vi "ON-OFF Cycle Timer - msec (SubVI).vi"(0 "ENABLE OUTPUT":bool, 5 "START/RESET":bool, 7 "ON Time [ms]":u32=10, 9 "OFF Time [ms]":u32=10, 11 "Cycle Limit":i32=100 min=-1) -> (4 "OUTPUT":bool, 6 "Cycle Change":bool, 8 "Cycles Complete":bool, 10 "Total Elapsed Time [ms]":u32, 14 "Display":string, 15 "Cycle Count":i32)   [LabVIEW 2012]
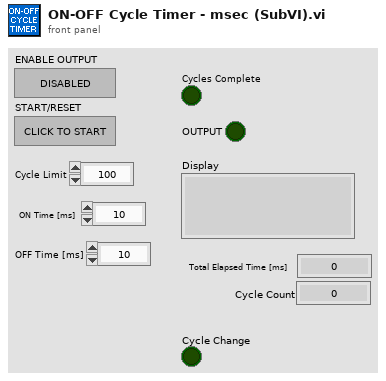
[diagram p1: front panel]
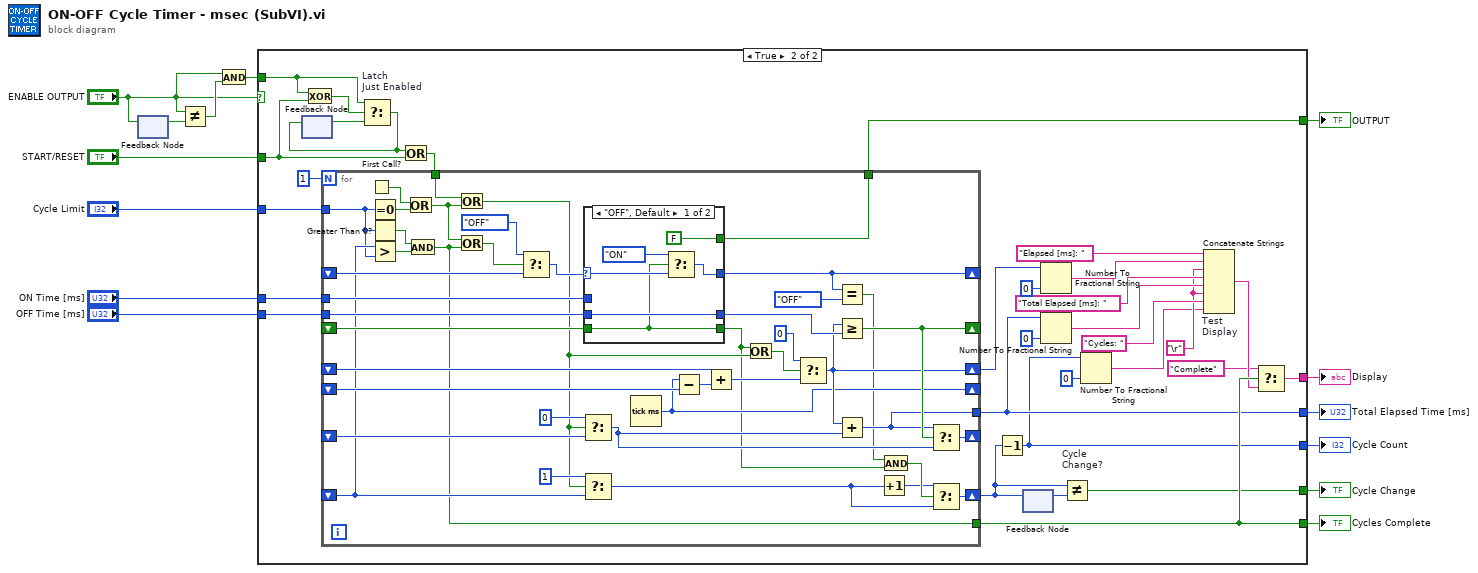
[diagram p0: block diagram]
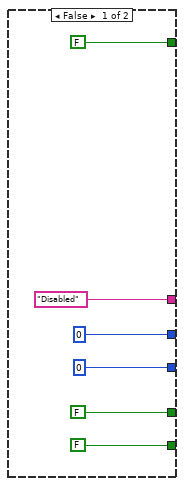
[diagram p2: hidden frame]
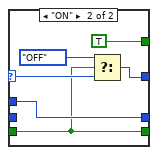
[diagram p3: hidden frame]
diagram:
  n1 = feedback #1() -> (w10:bool)  [unwired: 1 in]
  n2 = feedback-in #1("ENABLE OUTPUT") -> ()
  n3 = Not Equal?(x="ENABLE OUTPUT", y=w10) -> (x != y?=w12:bool)
  n4 = And(x="ENABLE OUTPUT", y=w12) -> (x .and. y?=w13:bool)
  n5 = case shown="True" "ENABLE OUTPUT" {
    tunnel: "ON Time [ms]" -> [_ w51]
    tunnel: "OFF Time [ms]" -> [_ w50]
    tunnel: [FALSE w38] -> w3
    tunnel: [FALSE w33] -> w4
    tunnel: [u32 0 w32] -> w5
    tunnel: [0 w31] -> w6
    tunnel: "Cycle Limit" -> [_ w28]
    tunnel: [FALSE w30] -> w8
    tunnel: ["Disabled" w29] -> w9
    tunnel: w13 -> [_ w25]
    tunnel: "START/RESET" -> [_ w23]
    frame False {
    }
    frame True {
      w41 = "\r"
      n6 = feedback #2() -> (w27:bool)  [unwired: 1 in]
      n7 = Exclusive Or(1:w23, 2:w25) -> (0:w26:bool)
      n8 = Select "Latch\nJust Enabled"(t=w25, s=w26, f=w27) -> (s? t:f=w24:bool)
      n9 = feedback-in #2(w24) -> ()
      n10 = Or(x=w24, y=w23) -> (x .or. y?=w22:bool)
      n11 = for {
        N: 1 -> [_]
        shift-right: [w78] -> _
        shift-left: _ -> [w93]
        shift-right: [w66] -> _
        shift-left: _ -> [w90]
        tunnel: w51 -> [w73]
        tunnel: w50 -> [w72]
        tunnel: [w91] -> w30
        shift-right: [w85] -> w34
        shift-left: _ -> [w61]
        shift-right: [w77] -> w39
        shift-left: _ -> [w83]
        shift-right: [w62] -> _
        shift-left: _ -> [w82]
        shift-right: [w70] -> _
        shift-left: _ -> [w74]
        tunnel: [w67] -> w32
        tunnel: [w55] -> w38
        tunnel: w28 -> [w60]
        tunnel: w22 -> [w56]
        n12 = First Call?() -> (First Call?: T/F=w58:bool)
        n13 = Equal To 0?(x=w60) -> (x = 0?=w59:bool)
        n14 = Greater Than 0?(x=w60) -> (x > 0?=w69:bool)
        n15 = Greater?(x=w61, y=w60) -> (0:w68:bool)
        n16 = Or(x=w58, y=w59) -> (x .or. y?=w54:bool)
        n17 = And(x=w69, y=w68) -> (x .and. y?=w55:bool)
        n18 = Or(x=w56, y=w54) -> (x .or. y?=w63:bool)
        n19 = Or(x=w54, y=w55) -> (x .or. y?=w71:bool)
        n20 = Select(t=enum16{"OFF", "ON"}."OFF" ("Mode (Read)"), s=w71, f=w90) -> (s? t:f=w65:enum16{"OFF", "ON"})
        n21 = Select(t=u32 0, s=w63, f=w74) -> (s? t:f=w75:u32)
        n22 = Select(t=1, s=w63, f=w61) -> (s? t:f=w86:i32)
        n23 = case shown="\"OFF\", Default" w65 {
          selector: w65 -> [w97 w103]
          tunnel: w93 -> [w95 w101]
          tunnel: [w98 w104] -> w66
          tunnel: w73 -> [_ w102]
          tunnel: [w96 w102] -> w92
          tunnel: w72 -> [w96 _]
          tunnel: [w95 w101] -> w53
          tunnel: [FALSE TRUE] -> w91
          frame "OFF", Default {
            n24 = Select(t=enum16{"OFF", "ON"}."ON" ("Mode (Read)"), s=w95, f=w97) -> (s? t:f=w98:enum16{"OFF", "ON"})
          }
          frame "ON" {
            n25 = Select(t=enum16{"OFF", "ON"}."OFF" ("Mode (Read)"), s=w101, f=w103) -> (s? t:f=w104:enum16{"OFF", "ON"})
          }
        }
        n26 = Tick Count (ms)() -> (millisecond timer value=w62:u32)
        n27 = Subtract(x=w62, y=w82) -> (x-y=w81:u32)
        n28 = Add(x=w83, y=w81) -> (x+y=w80:u32)
        n29 = Or(x=w53, y=w63) -> (x .or. y?=w64:bool)
        n30 = Select(t=u32 0, s=w64, f=w80) -> (s? t:f=w77:u32)
        n31 = Equal?(x=w66, y=enum16{"OFF", "ON"}."OFF") -> (x = y?=w52:bool)
        n32 = Greater Or Equal?(x=w77, y=w92) -> (x >= y?=w78:bool)
        n33 = Add(x=w77, y=w75) -> (x+y=w67:u32)
        n34 = Increment(x=w86) -> (x+1=w84:i32)
        n35 = And(x=w52, y=w53) -> (x .and. y?=w88:bool)
        n36 = Select(t=w67, s=w78, f=w75) -> (s? t:f=w70:u32)
        n37 = Select(t=w84, s=w88, f=w86) -> (s? t:f=w85:i32)
      }
      n38 = Decrement(x=w34) -> (x-1=w31:i32)
      n39 = feedback #3() -> (w35:i32)  [unwired: 1 in]
      n40 = feedback-in #3(w34) -> ()
      n41 = Number To Fractional String ("State Elapsed")(number=w39, precision (6)=i16 0) -> (F-format string=w46:string)  [unwired: 2 in]
      n42 = Number To Fractional String ("Total Elapsed")(number=w32, precision (6)=i16 0) -> (F-format string=w43:string)  [unwired: 2 in]
      n43 = Not Equal? "Cycle\nChange?"(x=w34, y=w35) -> (x != y?=w33:bool)
      n44 = Number To Fractional String ("Cycle Count")(number=w31, precision (6)=i16 0) -> (F-format string=w40:string)  [unwired: 2 in]
      n45 = Concatenate Strings "Test\nDisplay"("Elapsed [ms]: " ("string"), w46, w41, "Total Elapsed [ms]: " ("string"), w43, w41, "Cycles: " ("string"), w40) -> (w37:string)
      n46 = Select(t="Complete", s=w38, f=w37) -> (s? t:f=w29:string)
    }
  }
  "Cycle Count" <- w6
  "Total Elapsed Time [ms]" <- w5
  "Cycles Complete" <- w3
  "Display" <- w9
  "Cycle Change" <- w4
  "OUTPUT" <- w8
